vi "Get PTU File Frame Number.vi"(8 "error in (no error)":errorcluster, 11 "File Path":path) -> (0 "Error Out":errorcluster, 2 "Frame Start Indices":i32[](array[numeric]), 3 "# Frames":i32, 4 "Time (s)":dbl)   [LabVIEW 2021, in "PTU Files.lvlib"]
uses:
  PTU Files.lvlib
  Time/Time.lvlib
  PicoQuant.lvlib
  Utilities/Utilities.lvlib
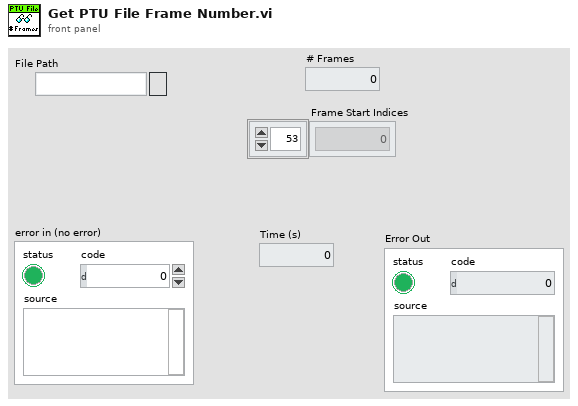
[diagram p1: front panel]
types:
  T1 = enum16{"big-endian, network order", "native, host order", "little-endian"}
  T2 = typedef "PTU Files.lvlib/PicoQuant Data File Information.ctl" = cluster{"PQ File Information":T3, "PQ Software Information":T4, "PQ Remote Request Information":T5, "PQ Hardware Information":T6, "PQ Measurement Information":T11, "PQ Image Information":T12, "PQ TT Results Format Information":T13, "PQ Measurement Results":T14}
  T3 = typedef "PTU Files.lvlib/PicoQuant File Information.ctl" = cluster{"GUID":string, "Assured Content":string, "Measurement Mode":i64, "Measurement SubMode":i64, "Comment":string, "Creation Time":string}
  T4 = typedef "PTU Files.lvlib/PicoQuant Software Information.ctl" = cluster{"Content Version":string, "Name":string, "Version":string, "# Modules":i64, "Module Names":string[], "Module Versions":string[], "SVN Build":i64}
  T5 = typedef "PTU Files.lvlib/PicoQuant Remote Request Information.ctl" = cluster{"Started by Remote Interface":bool, "Measurement Type":i64, "# Pixel X":i64, "# Pixel Y":i64, "Record Version":i64, "Scanning Pattern":i64, "Scanning Resolution (m/px)":dbl, "Comment":string, "File Name":string, "Group Name":string}
  T6 = typedef "PTU Files.lvlib/PicoQuant Hardware Information.ctl" = cluster{"Input Channels":T7, "Markers":T8, "Modules":T9, "Router Channels":T10}
  T7 = typedef "PTU Files.lvlib/PicoQuant Input Channels.ctl" = cluster{"# Input Channels":i64, "CFD Levels (mV)":i64[], "CFD Zero Crossings (mV)":i64[], "CFD Channel Enabled":bool[], "Module Indices":i64[], "Offsets (ps)":i64[], "Td Codes":i64[], "Trigger Edges":i64[], "Trigger Levels (mV)":i64[]}
  T8 = typedef "PTU Files.lvlib/PicoQuant Markers.ctl" = cluster{"# Markers":i64, "Markers Enabled":bool[], "Holdoff (ns)":i64, "Rising Edges":bool[]}
  T9 = typedef "PTU Files.lvlib/PicoQuant Modules.ctl" = cluster{"# Modules":i64, "Type Codes":i64[], "Version Codes":i64[]}
  T10 = typedef "PTU Files.lvlib/PicoQuant Router Channels.ctl" = cluster{"# Router Channels":i64, "CFD Levels (mV)":i64[], "CFD Present":bool[], "CFD Zero Crossings (mV)":i64[], "Input Levels (mV)":i64[], "Input Types":i64[], "Offsets (ps)":i64[], "Rising Edges":bool[], "Router Enabled":bool, "Router Model Code":i64, "Router Version":string, "Sync CFD Level (mV)":i64, "Sync CFD Zero Crossing (mV)":i64, "Sync Divider":i64, "Sync Offset (ps)":i64, "Sync Trigger Edge":i64, "Sync Trigger Level (mV)":i64, "Trigger Out On":bool, "Trigger Out Period (s)":dbl, "Base Resolution (s)":dbl, "External Devices":i64, "External Reference Clock":bool, "Features":u64, "Part Number":string, "Serial Number (string)":string, "Serial Number":i64, "Timing Mode":i64, "Hardware Type":string, "Hardware Version":string}
  T11 = typedef "PTU Files.lvlib/PicoQuant Measurement Information.ctl" = cluster{"Acquisition Time (ms)":i64, "Binning Factor":i64, "Global Resolution (s)":dbl, "Invalid Sync":bool, "Offset (ns)":u64, "# Curve Parameters":u64, "Devices":string[], "Names":string[], "Start Values":dbl[], "Steps":dbl[], "Stop Values":dbl[], "Tag Names":string[], "Units":string[], "Resolution (s)":dbl, "Restart":bool, "Stop At":u64, "Stop on Over f1":bool}
  T12 = typedef "PTU Files.lvlib/PicoQuant Image Information.ctl" = cluster{"Hardware Acceleration":i64, "Bidirectional":bool, "Dimensions":i64, "Frame Marker":i64, "Scanner Identity":i64, "Learning Time (s)":i64, "Line Frequency":dbl, "Line Start Marker":i64, "Line Stop Marker":i64, "Max Frames":i64, "Objective Name":string, "Pixel Resolution (um)":dbl, "# Pixels X":i64, "# Pixels Y":i64, "Preview Pixels/Line":i64, "Scan Direction":i64, "Sinusoidal Correction":i64, "Time per Line (ms)":dbl, "Time per Pixel (ms)":i64, "Velocity":i64, "X0 (um)":dbl, "X1 (um)":dbl, "X Calibration Offset (V)":dbl, "X Calibration (m/V)":dbl, "Y0 (um)":dbl, "Y1 (um)":dbl, "Y Calibration Offset (V)":dbl, "Y Calibration (m/V)":dbl, "Z0 (um)":dbl, "Z1 (um)":dbl, "Z Calibration Offset (V)":dbl, "Z  Calibration (m/V)":dbl}
  T13 = typedef "PTU Files.lvlib/PicoQuant Results Format.ctl" = cluster{"Bits per Record":i64, "Channel Mask":i64, "Channel Shift ":i64, "DTime Mask":i64, "DTime Shift":i64, "Marker Mask":i64, "Marker Shift":i64, "NSync Mask":i64, "NSync Shift":i64, "Special Mask":i64, "TTTR Record Type":i64, "Wrap Around":i64}
  T14 = typedef "PTU Files.lvlib/PicoQuant Measurement Results.ctl" = cluster{"Stop Reason":i64, "Input Rates (cps)":i64[], "Warning Flags":u64, "# Records":i64, "Stop After (ms)":i64, "Sync Rate (cps)":i64}
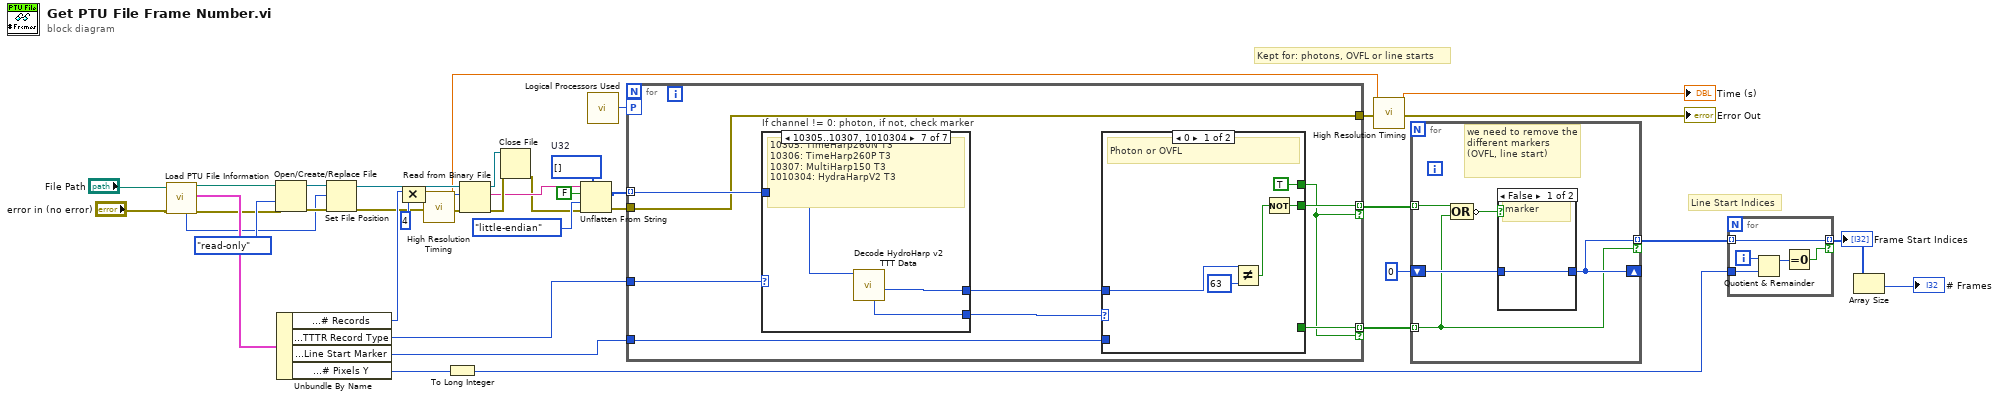
[diagram p0: block diagram]
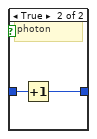
[diagram p2: hidden frame]
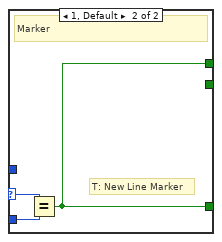
[diagram p3: hidden frame]
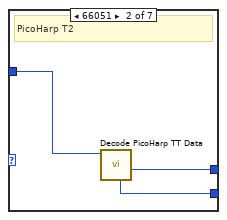
[diagram p5: hidden frame]
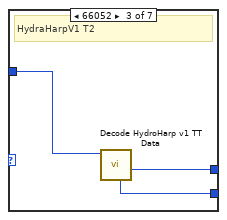
[diagram p6: hidden frame]
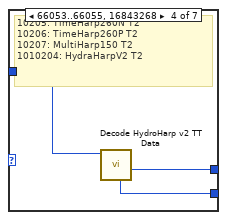
[diagram p7: hidden frame]
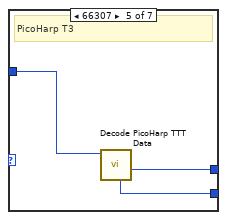
[diagram p8: hidden frame]
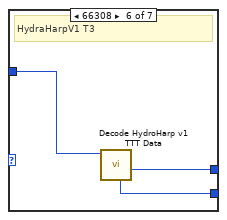
[diagram p9: hidden frame]
diagram:
  w33 = u32[] []  # U32
  # "Line Start Indices"
  # "Kept for: photons, OVFL or line starts"
  n1 = call "Load PTU File Information.vi"("error in (no error)"="error in (no error)", "File Path"="File Path") -> ("error out"=w21:errorcluster, "PicoQuant Data File Information"=w25:T2, "path (dup)"=w20:path, "Data offset (in bytes)"=w19:i64)  [unwired: 2 in, 4 out]
  n2 = Open/Create/Replace File(file path (use dialog)=w20, error in=w21, access (0:read/write)=enum16{"read/write", "read-only", "write-only"}."read-only") -> (refnum out=w22:refnum<file>, error out=w24:errorcluster)  [unwired: 3 in, 1 out]
  n3 = Unbundle By Name(w25) -> ("PQ Measurement Results.# Records"=w39:i64, "PQ TT Results Format Information.TTTR Record Type"=w6:i64, "PQ Image Information.Line Start Marker"=w5:i64, "PQ Image Information.# Pixels Y"=w28:i64)
  n4 = Set File Position(offset (in bytes) (0)=w19, refnum=w22, error in=w24) -> (refnum out=w17:refnum<file>, error out=w18:errorcluster)  [unwired: 1 in]
  n5 = Compound Arithmetic op=MULTIPLY(w39, i64 4) -> (w37:i64)
  n6 = call "High Resolution Timing.vi"("Error In"=w18) -> ("elapsed (relative) seconds"=w7:dbl, "Error Out"=w30:errorcluster)  [unwired: 16 in, 1 out]
  n7 = To Long Integer(number=w28) -> (32bit integer=w4:i32)
  n8 = Read from Binary File(8:w30, 10:w37, 11:w17) -> (0:w35:errorcluster, 2:w34:string, 3:w36:refnum<file>)  [unwired: 3 in, 1 out]
  n9 = Close File(refnum=w36, error in=w35) -> (error out=w29:errorcluster)  [unwired: 1 out]
  n10 = Unflatten From String(type=w33, binary string=w34, data includes array or string size? (T)=FALSE, byte order (0:big-endian, network order)=T1."little-endian", error in (no error)=w29) -> (value=w9:u32[], error out=w8:errorcluster)  [unwired: 1 out]
  n11 = call "Logical Processors Used.vi"() -> ("# Logical Processor Used"=w3:i32)  [unwired: 6 in]
  n12 = for {
    tunnel: w6 -> [w48]
    tunnel: w5 -> [w45]
    tunnel: w9 -> [w44] mode=indexing
    tunnel: w8 -> [w43]
    tunnel: [w43] -> w15
    tunnel: [w42] -> w13 mode=indexing if=w40
    tunnel: [w41] -> w12 mode=indexing if=w40
    workers-P: w3 -> [_]
    n13 = case "If channel != 0: photon, if not, check marker" shown="10305..10307, 1010304" w48 {
      tunnel: [_ w58 w60 w63 w67 w70 w72] -> w47
      tunnel: [_ w57 w61 w64 w68 w69 w73] -> w46
      tunnel: w44 -> [_ w59 w62 w65 w66 w71 w74]
      frame Default {
        # "unknown record type"
      }
      frame 66051 {
        # "PicoHarp T2"
        n14 = call "Decode PicoHarp TT Data.vi"("rawbits"=w59) -> ("channel"=w57:u8, "markercode"=w58:u32)  [unwired: 7 in, 2 out]
      }
      frame 66052 {
        # "HydraHarpV1 T2"
        n15 = call "Decode HydroHarp v1 TT Data.vi"("rawbits"=w62) -> ("channel"=w61:u8, "markercode"=w60:u32)  [unwired: 7 in, 2 out]
      }
      frame 66053..66055, 16843268 {
        # "10205: TimeHarp260N T2\n10206: TimeHarp260P T2 \n10207: MultiHarp150 T2\n1010204: HydraHarpV2 T2"
        n16 = call "Decode HydroHarp v2 TT Data.vi"("rawbits"=w65) -> ("channel"=w64:u8, "markercode"=w63:u32)  [unwired: 7 in, 2 out]
      }
      frame 66307 {
        # "PicoHarp T3"
        n17 = call "Decode PicoHarp TTT Data.vi"("rawbits"=w66) -> ("channel"=w68:u8, "markercode"=w67:u32)  [unwired: 6 in, 3 out]
      }
      frame 66308 {
        # "HydraHarpV1 T3"
        n18 = call "Decode HydroHarp v1 TTT Data.vi"("rawbits"=w71) -> ("channel"=w69:u8, "markercode"=w70:u32)  [unwired: 6 in, 3 out]
      }
      frame 66309..66311, 16843524 {
        # "10305: TimeHarp260N T3\n10306: TimeHarp260P T3\n10307: MultiHarp150 T3\n1010304: HydraHarpV2 T3"
        n19 = call "Decode HydroHarp v2 TTT Data.vi"("rawbits"=w74) -> ("channel"=w73:u8, "markercode"=w72:u32)  [unwired: 6 in, 3 out]
      }
    }
    n20 = case shown="0" w47 {
      selector: w47 -> [_ w56]
      tunnel: w46 -> [w53 _]
      tunnel: w45 -> [_ w55]
      tunnel: [TRUE w54] -> w40
      tunnel: [_ w54] -> w42
      tunnel: [w49 _] -> w41
      frame 0 {
        # "Photon or OVFL"
        n21 = Not Equal?(x=w53, y=u8 63) -> (x != y?=w50:bool)
        n22 = Not(x=w50) -> (.not. x?=w49:bool)
      }
      frame 1, Default {
        # "T: New Line Marker"
        # "Marker"
        n23 = Equal?(x=w56, y=w55) -> (x = y?=w54:bool)
      }
    }
  }
  n24 = call "High Resolution Timing.vi"("relative seconds (NaN)"=w7, "Error In"=w15) -> ("elapsed (relative) seconds"=→"Time (s)":dbl, "Error Out"=→"Error Out":errorcluster)  [unwired: 15 in, 1 out]
  n25 = for {
    tunnel: w13 -> [w75] mode=indexing
    tunnel: w12 -> [w79] mode=indexing
    shift-right: [w76] -> _
    shift-left: 0 -> [w77]
    tunnel: [w76] -> w10 mode=indexing if=w75
    # "we need to remove the different markers (OVFL, line start)"
    n26 = Compound Arithmetic op=OR(w79, w75) -> (invert w78:bool)
    n27 = case shown="False" w78 {
      tunnel: w77 -> [w80 w82]
      tunnel: [w80 w81] -> w76
      frame False {
        # "marker"
      }
      frame True {
        # "photon"
        n28 = Increment(x=w82) -> (x+1=w81:i32)
      }
    }
  }
  n29 = for {
    tunnel: w10 -> [w85] mode=indexing
    tunnel: w4 -> [w87]
    tunnel: [w85] -> w2 mode=indexing if=w84
    i -> [w83]
    n30 = Quotient & Remainder(x=w83, y=w87) -> (x-y*floor(x/y)=w86:i32)  [unwired: 1 out]
    n31 = Equal To 0?(x=w86) -> (x = 0?=w84:bool)
  }
  "Frame Start Indices" <- w2
  n32 = Array Size(array=w2) -> (size(s)=→"# Frames":i32)
